vi "buzzer.vi"() -> ()   [LabVIEW 2018]
uses:
  <vilib>/DAQmx/write.llb/DAQmx Write (Digital Bool 1Line 1Point).vi
  <vilib>/DAQmx/miscellaneous.llb/DAQmx Fill In Error Info.vi
panel:
  in  "True":bool
  in  "False":bool
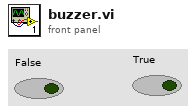
[diagram p1: front panel]
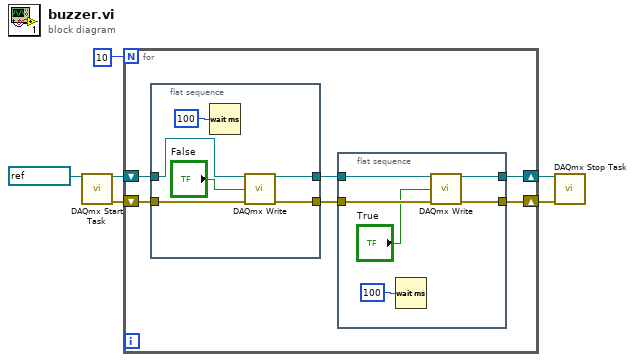
[diagram p0: block diagram]
diagram:
  n1 = call <vilib>:"DAQmx Start Task.vi"("task/channels in"=refnum<k21> "buzzer") -> ("task out"=w3:refnum<k21>, "error out"=w5:errorcluster)  [unwired: 13 in]
  n2 = for {
    N: 10 -> [_]
    shift-right: [w8] -> w6
    shift-left: w5 -> [w12]
    shift-right: [w7] -> w4
    shift-left: w3 -> [w11]
    n3 = flat-sequence {
      tunnel: w12 -> [w24]
      tunnel: w11 -> [w23]
      tunnel: [w21] -> w10
      tunnel: [w20] -> w9
      frame #0 {
        n4 = Wait (ms)(milliseconds to wait=u32 100) -> ()  [unwired: 1 out]
        n5 = call-poly <vilib>:"DAQmx Write.vi"("task/channels in"=w23, "data"="False", "error in"=w24) -> ("task out"=w21:refnum<k21>, "error out"=w20:errorcluster)  [unwired: 10 in, 1 out]
      }
    }
    n6 = flat-sequence {
      tunnel: w10 -> [w18]
      tunnel: w9 -> [w17]
      tunnel: [w16] -> w8
      tunnel: [w15] -> w7
      frame #0 {
        n7 = Wait (ms)(milliseconds to wait=u32 100) -> ()  [unwired: 1 out]
        n8 = call-poly <vilib>:"DAQmx Write.vi"("task/channels in"=w18, "data"="True", "error in"=w17) -> ("task out"=w15:refnum<k21>, "error out"=w16:errorcluster)  [unwired: 10 in, 1 out]
      }
    }
  }
  n9 = call <vilib>:"DAQmx Stop Task.vi"("task/channels in"=w4, "error in"=w6) -> ()  [unwired: 12 in, 2 out]
